vi "runExperiment.vi"(8 "error in (no error)":errorcluster, 10 "runExperiment":T1, 11 "ExperimentControl in":refnum<class "ExperimentControl.lvclass">) -> (0 "error out":errorcluster, 3 "ExperimentControl out":refnum<class "ExperimentControl.lvclass">)   [LabVIEW 2009, in "Views.lvlib" / "ExperimentControl.lvlib" / "ExperimentControl.lvclass"]
uses:
  ExperimentControl.lvclass
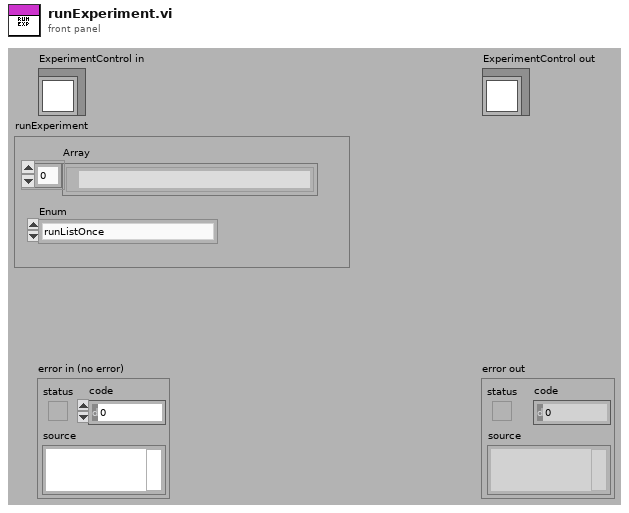
[diagram p1: front panel]
types:
  T1 = cluster{"Array":path[], "Enum":enum16{"runListOnce", "loopOverList"}}
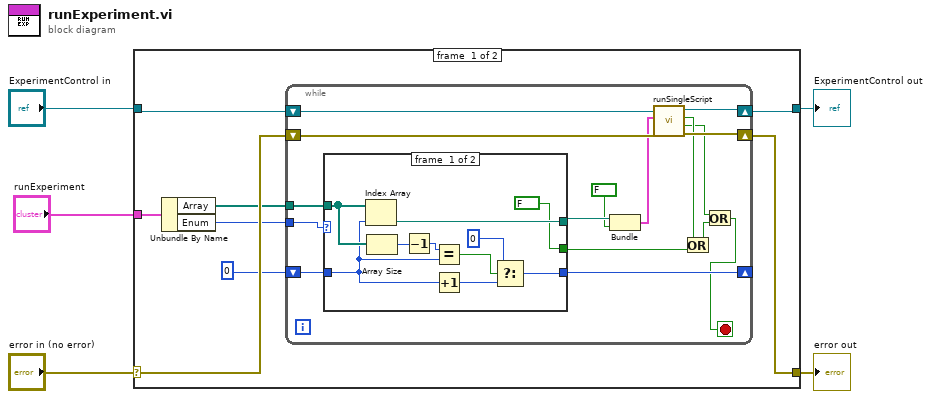
[diagram p0: block diagram]
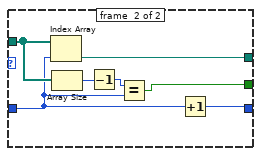
[diagram p2: hidden frame]
diagram:
  n1 = case shown="No Error" "error in (no error)" {
    selector: "error in (no error)" -> [w10 w48]
    tunnel: [w9 w48] -> w4
    tunnel: [w11 w47] -> w2
    tunnel: "ExperimentControl in" -> [w12 w47]
    tunnel: "runExperiment" -> [w13 _]
    frame #0 {
      n2 = Unbundle By Name(w13) -> ("Array"=w8:path[], "Enum"=w7:enum16{"runListOnce", "loopOverList"})
      n3 = while {
        shift-right: [w28] -> w11
        shift-left: w12 -> [w29]
        shift-right: [w26] -> w9
        shift-left: w10 -> [w27]
        tunnel: w8 -> [w25]
        tunnel: w7 -> [w24]
        shift-right: [w23] -> _
        shift-left: 0 -> [w22]
        stop <- w14 stop-if-true
        n4 = case shown="\"loopOverList\"" w24 {
          tunnel: w25 -> [w38 w45]
          tunnel: [w39 w46] -> w21
          tunnel: [w31 w42] -> w23
          tunnel: w22 -> [w33 w40]
          tunnel: [FALSE w41] -> w17
          frame #0 {
            n5 = Index Array(array=w38, index=w33) -> (element=w39:path)
            n6 = Array Size(array=w38) -> (size(s)=w36:i32)
            n7 = Decrement(x=w36) -> (x-1=w37:i32)
            n8 = Equal?(x=w37, y=w33) -> (x = y?=w35:bool)
            n9 = Increment(x=w33) -> (x+1=w30:i32)
            n10 = Select(t=0, s=w35, f=w30) -> (s? t:f=w31:i32)
          }
          frame #1 {
            n11 = Index Array(array=w45, index=w40) -> (element=w46:path)
            n12 = Array Size(array=w45) -> (size(s)=w43:i32)
            n13 = Decrement(x=w43) -> (x-1=w44:i32)
            n14 = Equal?(x=w44, y=w40) -> (x = y?=w41:bool)
            n15 = Increment(x=w40) -> (x+1=w42:i32)
          }
        }
        n16 = Bundle("Path"=w21, FALSE) -> (w19:cluster{"Path":path, bool})  [unwired: 1 in]
        n17 = call "runSingleScript.vi"("error in (no error)"=w27, "runSingleScript"=w19, "ExperimentControl in"=w29) -> ("error out"=w26:errorcluster, "stopBeforeNext"=w16:bool, "stoppedByUser"=w18:bool, "ExperimentControl out"=w28:refnum<class "ExperimentControl.lvclass">)  [unwired: 5 in]
        n18 = Or(x=w18, y=w17) -> (x .or. y?=w15:bool)
        n19 = Or(x=w16, y=w15) -> (x .or. y?=w14:bool)
      }
    }
    frame #1 {
    }
  }
  "error out" <- w4
  "ExperimentControl out" <- w2
